vi "WPI_CameraDecodeJPEGString.vi"(4 "error in":errorcluster, 6 "Compressed Image":string, 7 "Image In":T1) -> (0 "error out":errorcluster, 3 "Image Out":T1)   [LabVIEW 2017]
doc: "This software is licensed. Open the labview\\readme\\WPI Robotics Library Open Source License.txt file for more information."
uses:
  <vilib>/vision/Image Controls.llb/IMAQ Image.ctl
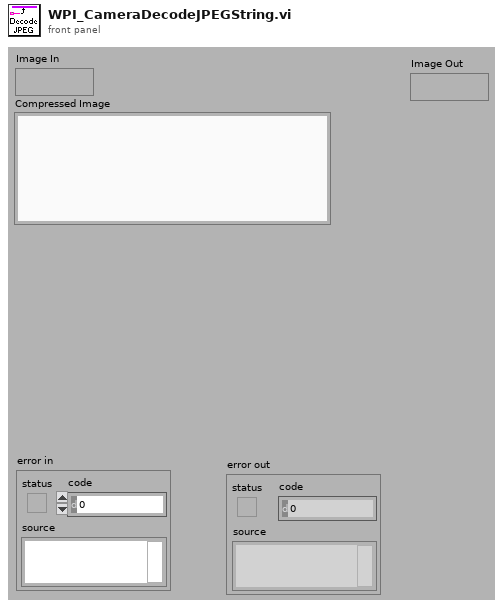
[diagram p1: front panel]
types:
  T1 = typedef "IMAQ Image.ctl" = refnum<image>
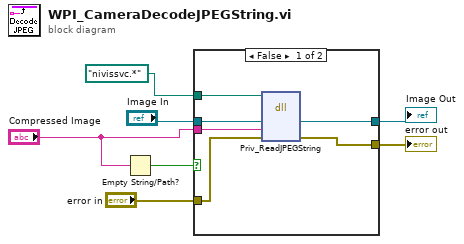
[diagram p0: block diagram]
diagram:
  n1 = Empty String/Path?(string/path="Compressed Image") -> (empty?=w2:bool)
  n2 = case shown="False" w2 {
    tunnel: "Compressed Image" -> [w13 _]
    tunnel: "Image In" -> [w12 w15]
    tunnel: "error in" -> [w11 w14]
    tunnel: [w10 w14] -> w5
    tunnel: [w9 w15] -> w4
    tunnel: path "nivissvc.*" ("path in") -> [w8 _]
    frame False {
      n3 = dll-call lib="nivissvc.*" fn="Priv_ReadJPEGString"(path in=w8, "image"=w12, "name"=w13, "err"=w11) -> ("image"=w9:T1, "err"=w10:errorcluster)  [unwired: 3 in, 3 out]
    }
    frame True {
    }
  }
  "error out" <- w5
  "Image Out" <- w4
